vi "Configure.vi"(8 "error in (no error)":errorcluster, 11 "AOTF in":refnum<class "AOTF.lvclass">) -> (0 "error out":errorcluster, 2 "cancelled?":bool, 3 "AOTF out":refnum<class "AOTF.lvclass">)   [LabVIEW 2012, in "AOTF.lvclass"]
doc: "The configure method configures the details for the RabbitMQ connection. \n\nIn the derived class, make a call to the parent for setting these parameters."
uses:
  AOTF.lvclass
  <vilib>/Utility/miscctls.llb/LVPointTypeDef.ctl
  <vilib>/Distrio/Murmex/Murmex/Murmex.lvclass
panel:
  in  "Tab Control":enum32{"Comport", "Debug"}(tab)
  in  "DO lines":tag
  in  "AO channel":tag
  in  "LUT561":path=path "D:/CLSM_Project/AOTF/561nm.txt" caption="LUT 561nm"
  in  "LUT515":path=path "D:/CLSM_Project/AOTF/515nm.txt" caption="LUT 515nm"
  in  "LUT491":path=path "D:/CLSM_Project/AOTF/491nm.txt" caption="LUT 491nm"
  in  "LUT445":path=path "D:/CLSM_Project/AOTF/445nm.txt" caption="LUT 445nm"
  in  "LUT405":path=path "D:/CLSM_Project/AOTF/405nm.txt" caption="LUT 405nm"
  in  "button::configure murmex":bool
  in  "button::ok":bool
  in  "button::cancel":bool
  # "RabbitMQ parameters"
  # "Window position"
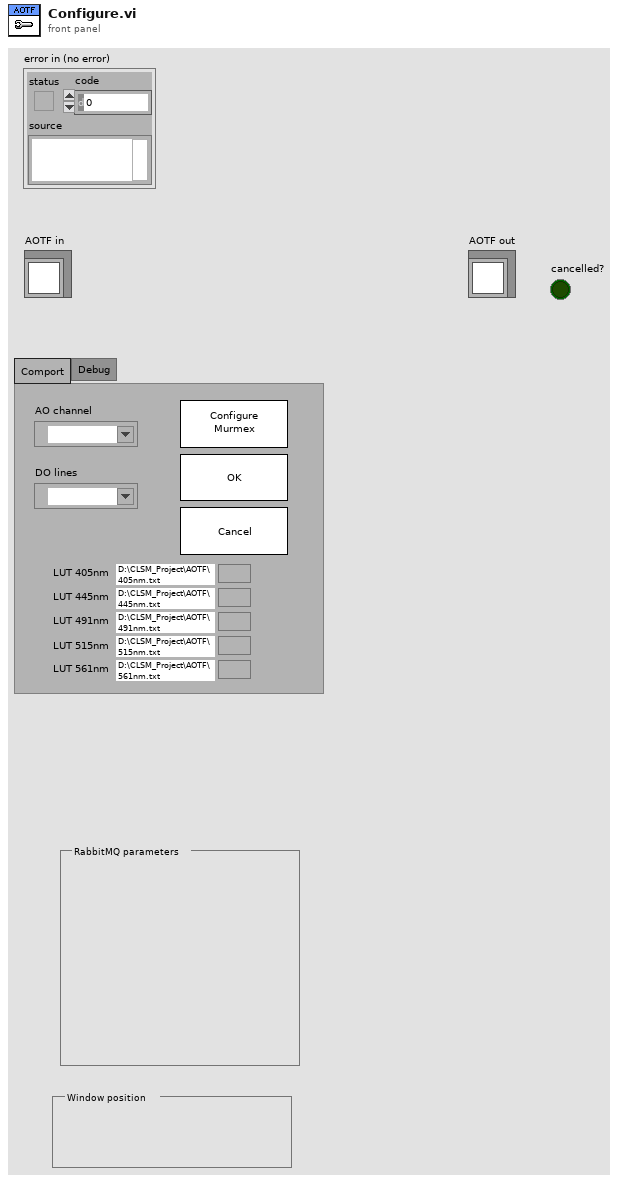
[diagram p1: front panel]
types:
  T1 = typedef "LVPointTypeDef.ctl" = cluster{"Horizontal":i16, "Vertical":i16}
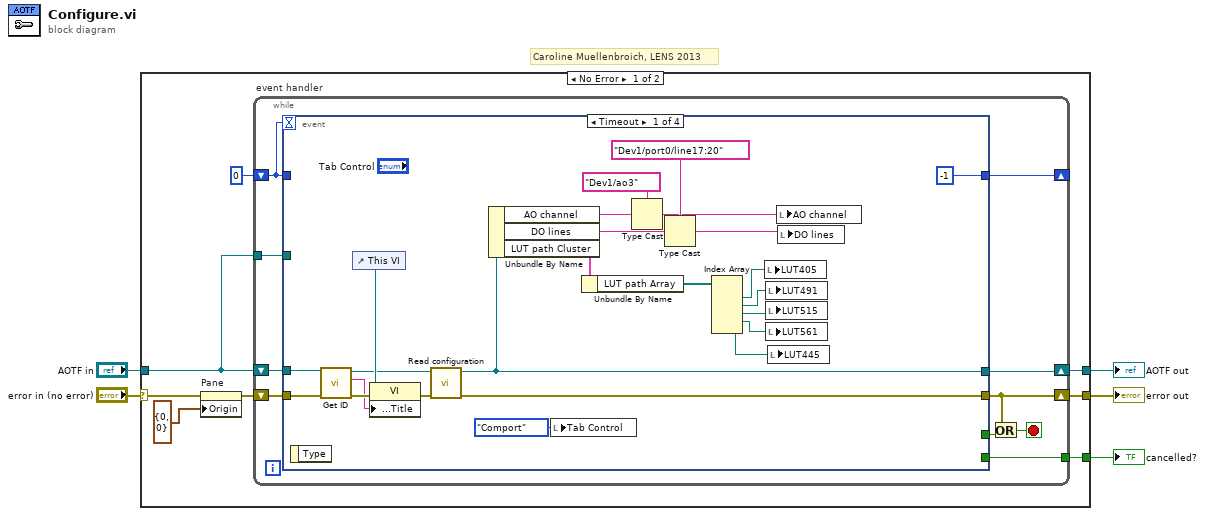
[diagram p0: block diagram]
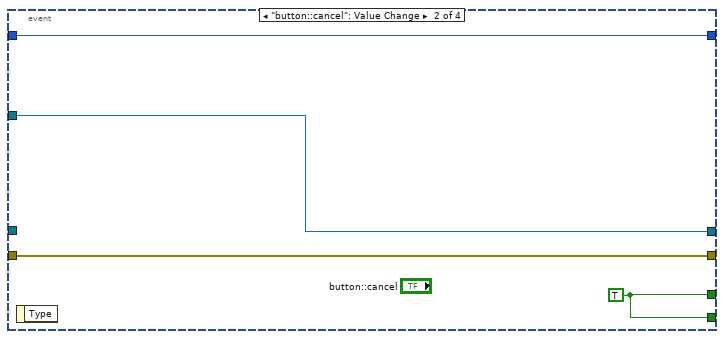
[diagram p2: hidden frame]
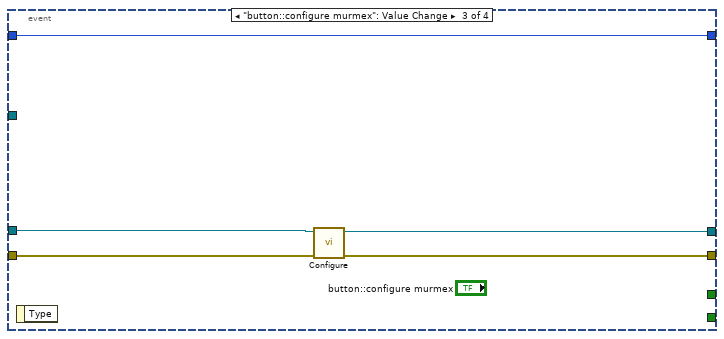
[diagram p3: hidden frame]
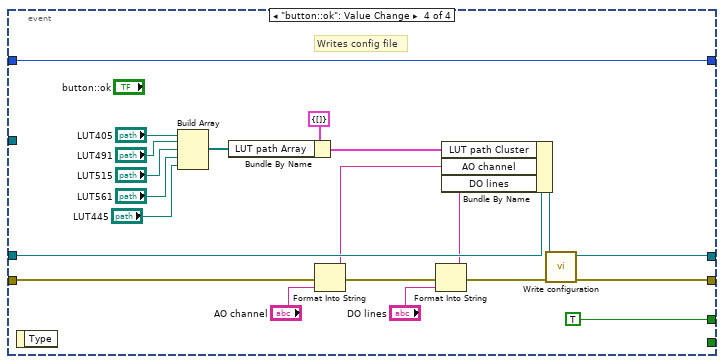
[diagram p4: hidden frame]
diagram:
  # "Caroline Muellenbroich, LENS 2013"
  n1 = case shown="No Error" "error in (no error)" {
    selector: "error in (no error)" -> [w11 w78]
    tunnel: "AOTF in" -> [w12 w79]
    tunnel: [w8 w78] -> w1
    tunnel: [w7 w79] -> w3
    tunnel: [w6 _] -> w2
    frame No Error {
      n2 = property on="Pane" class="Pane"(error in=w11, "Origin"=T1 {"Horizontal"=0, "Vertical"=0}) -> (error out=w10:errorcluster)  [unwired: 1 in, 1 out]
      n3 = while "event handler" {
        shift-right: [w23] -> _
        shift-left: 0 -> [w14]
        shift-right: [w19] -> w7
        shift-left: w12 -> [w22]
        tunnel: w12 -> [w21]
        shift-right: [w17] -> w8
        shift-left: w10 -> [w20]
        tunnel: [w15] -> w6
        stop <- w18 stop-if-true
        n4 = event shown="[0] Timeout" {
          selector: _ -> [_ _ _ _]
          dyn-events: _ -> [_ _ _ _]
          timeout: w14 -> [_ _ _ _]
          tunnel: w14 -> [_ w51 w56 w77]
          tunnel: [-1 w51 w56 w77] -> w23
          tunnel: w22 -> [w43 _ w53 w74]
          tunnel: w21 -> [_ w48 _ _]
          tunnel: w20 -> [w46 w49 w52 w68]
          tunnel: [w39 w48 w54 w75] -> w19
          tunnel: [w38 w49 w55 w76] -> w17
          tunnel: [_ w50 _ TRUE ("force loading?")] -> w16
          tunnel: [_ w50 _ _] -> w15
          event Timeout {
            n5 = event-data() -> ()  [unwired: 1 in, 1 out]
            n6 = call <vilib>:"Get ID.vi"("error in (no error)"=w46, "Murmex in"=w43) -> ("error out"=w44:errorcluster, "component id"=w42:string, "Murmex out"=w40:refnum<class "AOTF.lvclass">)  [unwired: 7 in]
            n7 = control-ref of="This VI"() -> (w45:refnum<vi>)
            n8 = property class="VI"(reference=w45, error in=w44, "Front Panel.Title"=w42) -> (error out=w41:errorcluster)  [unwired: 1 out]
            n9 = call <vilib>:"Read configuration.vi"("error in (no error)"=w41, "Murmex in"=w40) -> ("error out"=w38:errorcluster, "Murmex out"=w39:refnum<class "AOTF.lvclass">)  [unwired: 7 in, 1 out]
            n10 = Unbundle By Name(w39) -> ("AO channel"=w33:string, "DO lines"=w32:string, "LUT path Cluster"=w36:cluster{"LUT path Array":path[]})
            n11 = local write "Tab Control"(enum32{"Comport", "Debug"}."Comport" ("Tab Control")) -> ()
            n12 = Unbundle By Name(w36) -> ("LUT path Array"=w35:path[])
            n13 = Type Cast(type=tag "Dev1/ao3" ("AO channel"), x=w33) -> (*(type *) &x=w29:tag)
            n14 = Type Cast(type=tag "Dev1/port0/line17:20" ("DO lines"), x=w32) -> (*(type *) &x=w28:tag)
            n15 = Index Array(array=w35) -> (element #1=w34:path, element #2=w27:path, element #3=w26:path, element #4=w25:path, element #5=w24:path)  [unwired: 5 in]
            n16 = local write "LUT405"(w34) -> ()
            n17 = local write "LUT491"(w27) -> ()
            n18 = local write "LUT515"(w26) -> ()
            n19 = local write "LUT561"(w25) -> ()
            n20 = local write "LUT445"(w24) -> ()
            n21 = local write "AO channel"(w29) -> ()
            n22 = local write "DO lines"(w28) -> ()
          }
          event "button::cancel": Value Change {
            w50 = TRUE ("force loading?")
            n23 = event-data() -> ()  [unwired: 1 in, 1 out]
          }
          event "button::configure murmex": Value Change {
            n24 = event-data() -> ()  [unwired: 1 in, 1 out]
            n25 = call-parent "Configure.vi"("error in (no error)"=w52, "Murmex in"=w53) -> ("error out"=w55:errorcluster, "Murmex out"=w54:refnum<class "AOTF.lvclass">)  [unwired: 7 in, 1 out]
          }
          event "button::ok": Value Change {
            # "Writes config file"
            n26 = event-data() -> ()  [unwired: 1 in, 1 out]
            n27 = Build Array("LUT405", "LUT491", "LUT515", "LUT561", "LUT445") -> (w71:path[])
            n28 = Bundle By Name(cluster=cluster{"LUT path Array":path[]} {"LUT path Array"=[]} ("Confiugration cluster.LUT path Cluster"), "LUT path Array"=w71) -> (w61:cluster{"LUT path Array":path[]})
            n29 = Format Into String(error in=w68, "AO channel") -> (resulting string=w63:string, error out=w67:errorcluster)  [unwired: 2 in]
            n30 = Format Into String(error in=w67, "DO lines") -> (resulting string=w64:string, error out=w66:errorcluster)  [unwired: 2 in]
            n31 = Bundle By Name(cluster=w74, "LUT path Cluster"=w61, "AO channel"=w63, "DO lines"=w64) -> (w73:refnum<class "AOTF.lvclass">)
            n32 = call <vilib>:"Write configuration.vi"("error in (no error)"=w66, "Murmex in"=w73) -> ("error out"=w76:errorcluster, "Murmex out"=w75:refnum<class "AOTF.lvclass">)  [unwired: 8 in]
          }
        }
        n33 = Or(x=w17, y=w16) -> (x .or. y?=w18:bool)
      }
    }
    frame Error {
    }
  }
  "error out" <- w1
  "AOTF out" <- w3
  "cancelled?" <- w2
